vi "Detect Pulses in File.vi"(8 "Delay":dbl=0.013735 format="%#_6p", 9 "Channel name":string="CH0", 10 "RP I-V Configuration":T1={"I-V parameters"={"Start magnitude"=0.0, "Magnitude increment"=0.0, "End magnitude"=0.0, "Baseline length"=0, "Ramp length"=0, "Top  length"=0, "Threshold "=0.0, "Processing delay"=0, "Valhalla range"=0.0, "Interpolation"=0}, "Ranges"=[], "Pre-trigger duration"=0.01, "Post-trigger duration"=0.1, "Output delay"=0.1} {"Output delay" format="%#_6ps"; "Post-trigger duration" format="%#_6ps"; "Pre-trigger duration" format="%#_6ps"; "Ranges" format="%#_6pV"; "I-V parameters"."Valhalla range" format="%#_6pA"; "I-V parameters"."Processing delay" format="%dpts"; "I-V parameters"."Threshold" format="%#_6pV"; "I-V parameters"."Top  length" format="%dpts"; "I-V parameters"."Ramp length" format="%dpts"; "I-V parameters"."Baseline length" format="%dpts"; "I-V parameters"."End magnitude" format="%#_6pA"; "I-V parameters"."Magnitude increment" format="%#_6pA"; "I-V parameters"."Start magnitude" format="%#_6pA"}, 11 "File Path":path) -> (0 "Avg signal minus\nAvg background":dbl[](graph), 1 "Pulse indices out":T3[](array[typedef]), 2 "data":waveform(dbl), 4 "RP I-V Configuration out":T1={"I-V parameters"={"Start magnitude"=0.0, "Magnitude increment"=0.0, "End magnitude"=0.0, "Baseline length"=0, "Ramp length"=0, "Top  length"=0, "Threshold "=0.0, "Processing delay"=0, "Valhalla range"=0.0, "Interpolation"=0}, "Ranges"=[], "Pre-trigger duration"=0.01, "Post-trigger duration"=0.1, "Output delay"=0.1} {"Output delay" format="%#_6ps"; "Post-trigger duration" format="%#_6ps"; "Pre-trigger duration" format="%#_6ps"; "Ranges" format="%#_6pV"; "I-V parameters"."Valhalla range" format="%#_6pA"; "I-V parameters"."Processing delay" format="%dpts"; "I-V parameters"."Threshold" format="%#_6pV"; "I-V parameters"."Top  length" format="%dpts"; "I-V parameters"."Ramp length" format="%dpts"; "I-V parameters"."Baseline length" format="%dpts"; "I-V parameters"."End magnitude" format="%#_6pA"; "I-V parameters"."Magnitude increment" format="%#_6pA"; "I-V parameters"."Start magnitude" format="%#_6pA"})   [LabVIEW 2016]
uses:
  Pulse indexies.ctl
  RP Core/Rep Pitaya I-V driver/RP I-V Configuration.ctl
  I-V parameters.ctl
panel:
  in  "Skip 1st #points":i32
  out "Waveform Graph 2":dbl[][](graph)
  out "Waveform Graph":dbl[][](graph)
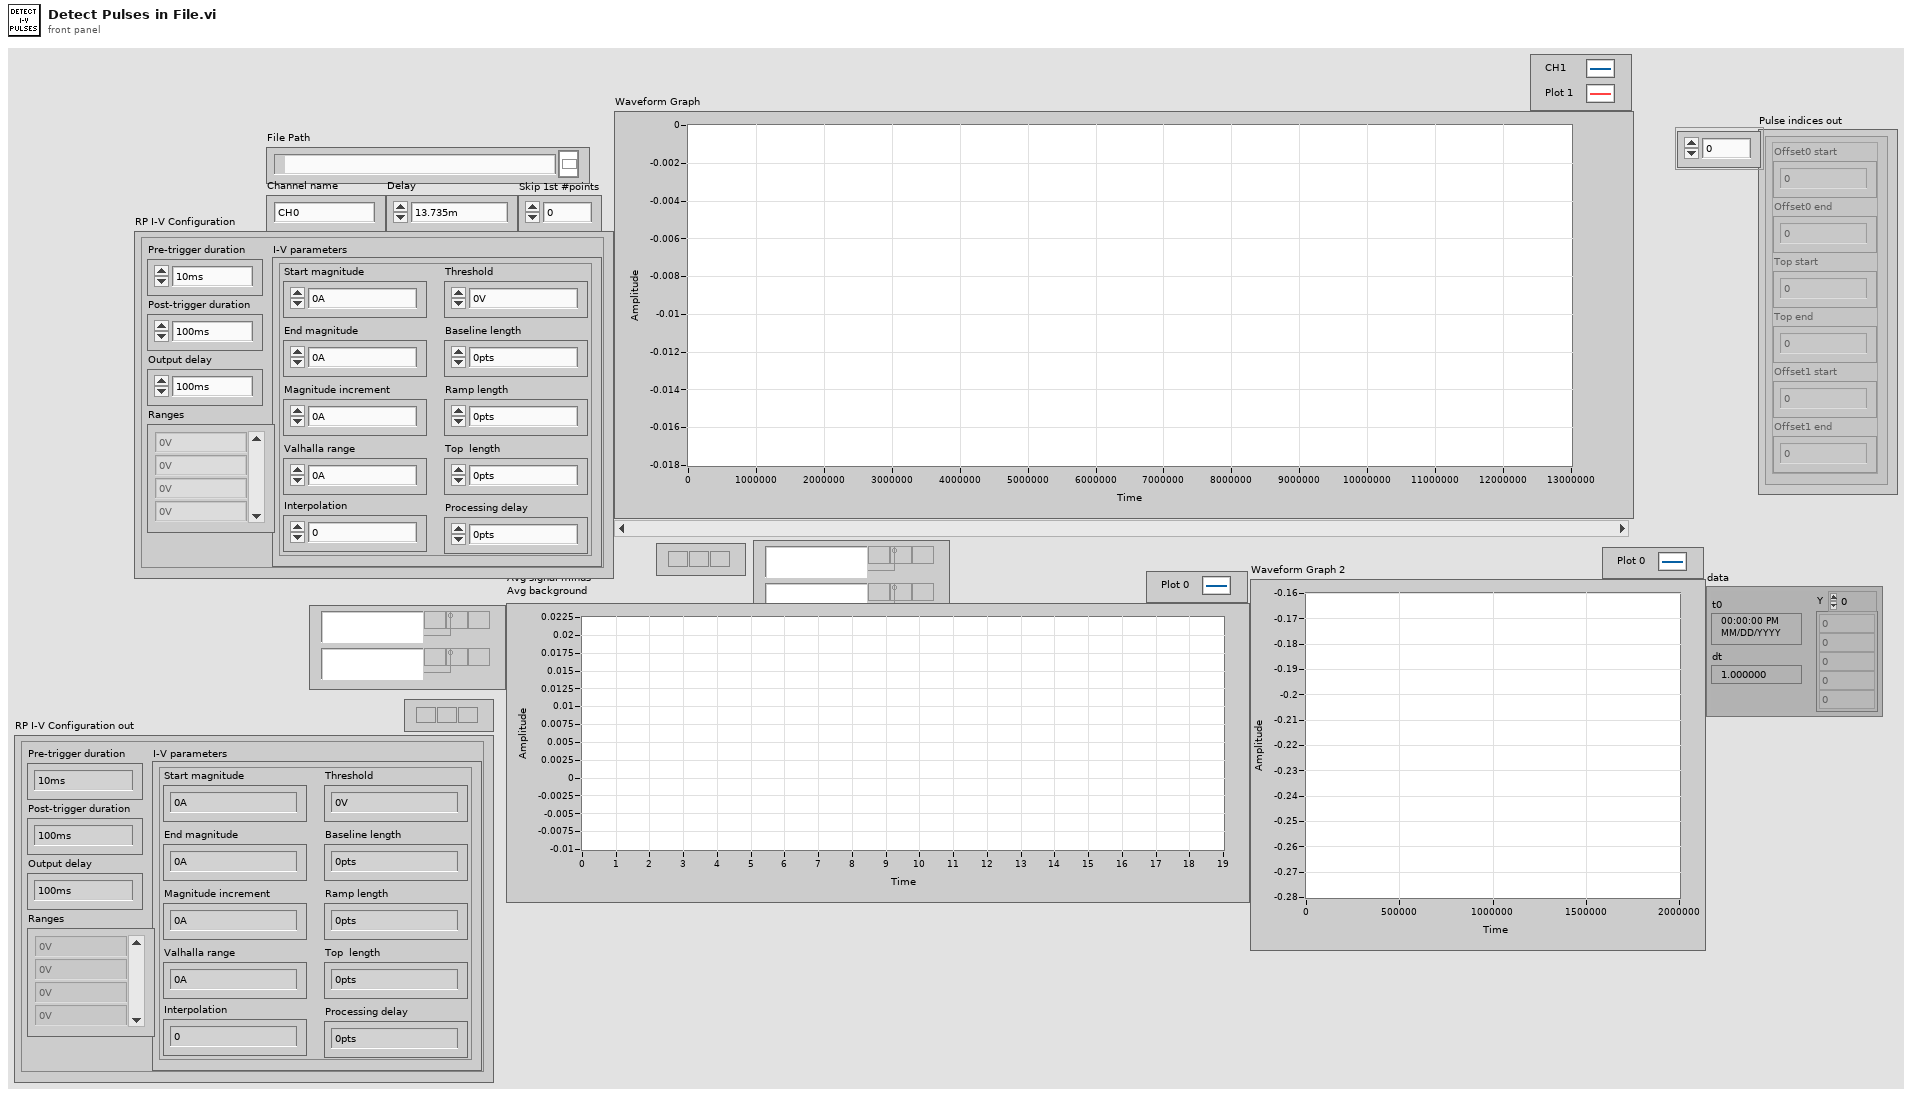
[diagram p1: front panel]
types:
  T1 = typedef "RP I-V Configuration.ctl" = cluster{"I-V parameters":T2, "Ranges":dbl[], "Pre-trigger duration":dbl, "Post-trigger duration":dbl, "Output delay":dbl}
  T2 = typedef "I-V parameters.ctl" = cluster{"Start magnitude":dbl, "Magnitude increment":dbl, "End magnitude":dbl, "Baseline length":i32, "Ramp length":i32, "Top  length":i32, "Threshold ":dbl, "Processing delay":u16, "Valhalla range":dbl, "Interpolation":i32}
  T3 = typedef "Pulse indexies.ctl" = cluster{"Offset0 start ":i32, "Offset0 end":i32, "Top start":i32, "Top end":i32, "Offset1 start":i32, "Offset1 end":i32}
  T4 = enum16{"open", "open or create", "create or replace", "create", "open (read-only)"}
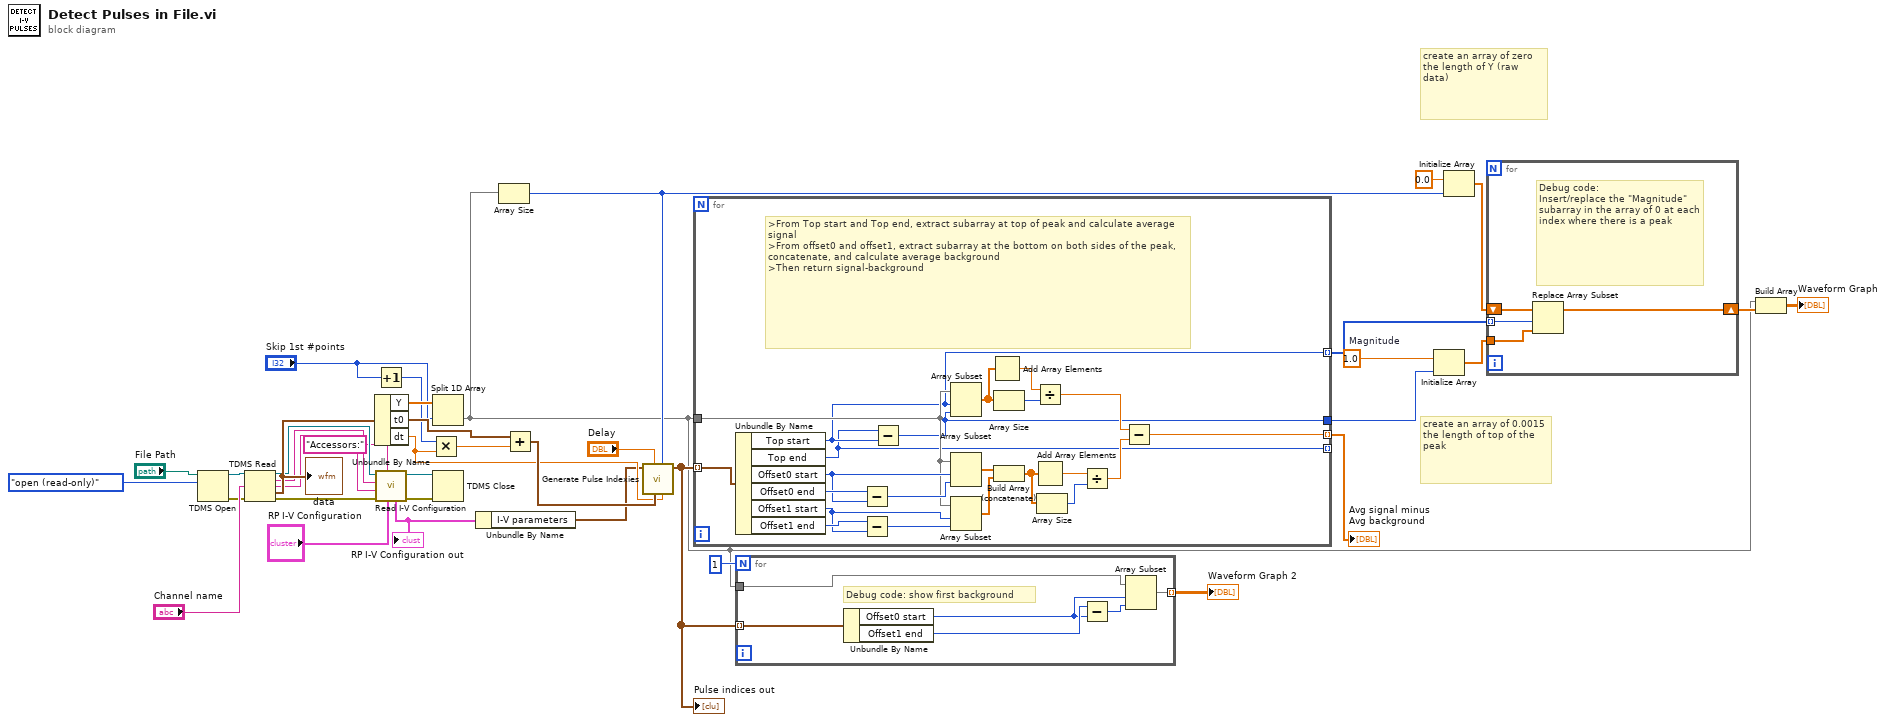
[diagram p0: block diagram]
diagram:
  w25 = 1.0  # Magnitude
  # "create an array of 0.0015 the length of top of the peak"
  # "create an array of zero the length of Y (raw data)"
  n1 = TDMS Open(10:T4."open (read-only)" ("operation (0:open)"), 11:"File Path") -> (0:w11:errorcluster, 3:w10:refnum<k34>)  [unwired: 5 in]
  n2 = TDMS Read(0:w10, 7:"Channel name", 11:w11) -> (4:w9:refnum<k34>, 6:w7:string, 8:w6:string, 10:w19:waveform(dbl), 15:w8:errorcluster)  [unwired: 5 in, 1 out]
  "data" <- w19
  n3 = Unbundle By Name(w19) -> ("Y"=w31:dbl[], "t0"=w35:timestamp, "dt"=w15:dbl)
  n4 = Increment(x="Skip 1st #points") -> (x+1=w13:i32)
  n5 = call "Read I-V Configuration.vi"("RP I-V Configuration in"="RP I-V Configuration", "Prefix"="Accessors:", "Error In"=w8, "channel name"=w6, "group name"=w7, "tdms file"=w9) -> ("Error Out"=w3:errorcluster, "tdms file out"=w2:refnum<k34>, "RP I-V Configuration out"=w5:T1)  [unwired: 3 out]
  "RP I-V Configuration out" <- w5
  n6 = Multiply(x=w13, y=w15) -> (x*y=w14:dbl)
  n7 = Split 1D Array(array=w31, index="Skip 1st #points") -> (second subarray=w18:dbl[])  [unwired: 1 out]
  n8 = TDMS Close(8:w3, 11:w2) -> ()  [unwired: 2 out]
  n9 = Unbundle By Name(w5) -> ("I-V parameters"=w4:T2)
  n10 = Array Size(array=w18) -> (size(s)=w28:i32)
  n11 = Add(x=w35, y=w14) -> (x+y=w17:timestamp)
  n12 = call "Generate Pulse Indexies.vi"("dt"=w15, "Size"=w28, "t0"=w17, "Delay"="Delay", "I-V parameters"=w4) -> ("Pulse indexies out"=w29:T3[])  [unwired: 6 in]
  "Pulse indices out" <- w29
  n13 = for {
    tunnel: w29 -> [w60] mode=indexing
    tunnel: w18 -> [w53]
    tunnel: [w43] -> w21 mode=indexing
    tunnel: [w41] -> w20 mode=indexing
    tunnel: [w40] -> _ mode=indexing
    tunnel: [w39] -> w26
    # ">From Top start and Top end, extract subarray at top of peak and calculate average signal\n>From offset0 and offset1, extract subarray at the bottom on both sides of the peak, concatenate, and calculate average background\n>Then return signal-background"
    n14 = Unbundle By Name(w60) -> ("Top start"=w41:i32, "Top end"=w40:i32, "Offset0 start"=w58:i32, "Offset0 end"=w59:i32, "Offset1 start"=w55:i32, "Offset1 end"=w56:i32)
    n15 = Subtract(x=w59, y=w58) -> (x-y=w57:i32)
    n16 = Subtract(x=w56, y=w55) -> (x-y=w54:i32)
    n17 = Subtract(x=w40, y=w41) -> (x-y=w39:i32)
    n18 = Array Subset(array=w53, index=w41, length=w39) -> (w50:dbl[])
    n19 = Array Subset(array=w53, index=w58, length=w57) -> (w52:dbl[])
    n20 = Array Subset(array=w53, index=w55, length=w54) -> (w51:dbl[])
    n21 = Add Array Elements(numeric array=w50) -> (sum=w49:dbl)
    n22 = Array Size(array=w50) -> (size(s)=w48:i32)
    n23 = Build Array (concatenate)(w52, w51) -> (w47:dbl[])
    n24 = Divide(x=w49, y=w48) -> (x/y=w44:dbl)
    n25 = Add Array Elements(numeric array=w47) -> (sum=w46:dbl)
    n26 = Array Size(array=w47) -> (size(s)=w45:i32)
    n27 = Divide(x=w46, y=w45) -> (x/y=w42:dbl)
    n28 = Subtract(x=w44, y=w42) -> (x-y=w43:dbl)
  }
  "Avg signal minus\nAvg background" <- w21
  n29 = for {
    N: 1 -> [_]
    tunnel: w29 -> [w65] mode=indexing
    tunnel: w18 -> [w66]
    tunnel: [w61] -> w32 mode=indexing
    # "Debug code: show first background"
    n30 = Unbundle By Name(w65) -> ("Offset0 start"=w63:i32, "Offset1 end"=w64:i32)
    n31 = Subtract(x=w64, y=w63) -> (x-y=w62:i32)
    n32 = Array Subset(array=w66, index=w63, length=w62) -> (w61:dbl[])
  }
  "Waveform Graph 2" <- w32
  n33 = Initialize Array(w25, w26) -> (w24:dbl[])
  n34 = Initialize Array(0.0, w28) -> (w27:dbl[])
  n35 = for {
    tunnel: w20 -> [w69] mode=indexing
    tunnel: w24 -> [w68]
    shift-right: [w67] -> w22
    shift-left: w27 -> [w70]
    # "Debug code:\nInsert/replace the \"Magnitude\" subarray in the array of 0 at each index where there is a peak"
    n36 = Replace Array Subset(array=w70, new element=w68, index=w69) -> (w67:dbl[])
  }
  n37 = Build Array(w18, w22) -> (→"Waveform Graph":dbl[][])
